vi "DIO_SPI.vi"(0 "DIO.2:0.OUT":fxp<+,3,3> format="%03b", 1 "DIO.2:0.DIR":fxp<+,3,3> format="%03b", 2 "SPI.CNT":u16, 3 "SPI.CNFG":u16 format="%016b", 4 "SPI.DATO":u16, 5 "SPI.GO":T1, 6 "DIO.2/SPI.MOSI Refnum":refnum<k21>, 7 "SELECT.1:0":fxp<+,2,2> format="%02b", 8 "DIO.1/SPI.MISO Refnum":refnum<k21>, 10 "DIO.0/SPI.SCLK Refnum":refnum<k21>) -> (14 "DIO.2:0.IN":fxp<+,3,3> format="%03b", 18 "SPI.DATI":u16, 19 "SPI.STAT":u8 format="%08b")   [LabVIEW 2015]
uses:
  Utilities/Start Boolean.ctl
panel:
  # "SELECT1 | SELECT0 || Functionality\n ---------|---------||------------------\n     0    |    0    || DIO0, DIO1, DIO2\n     0    |    1    || DIO1, SPI: MISO, SCLK (RX Only SPI)\n     1    |    0    || DIO0, SPI: MOSI, SCLK (TX Only SPI)\n     1    |    1    || SPI: MISO, MOSI, SCLK"
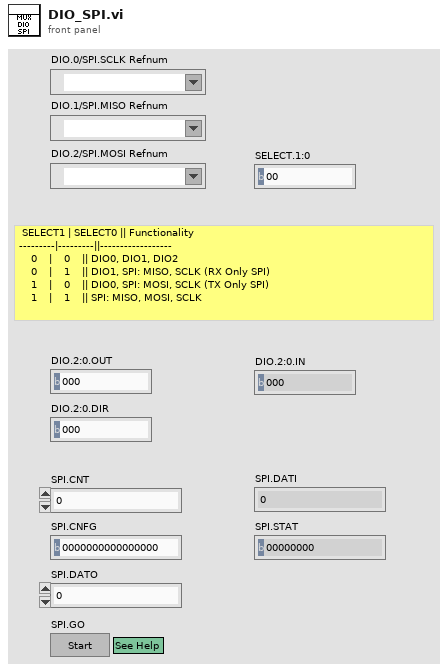
[diagram p1: front panel]
types:
  T1 = typedef "Start Boolean.ctl" = bool
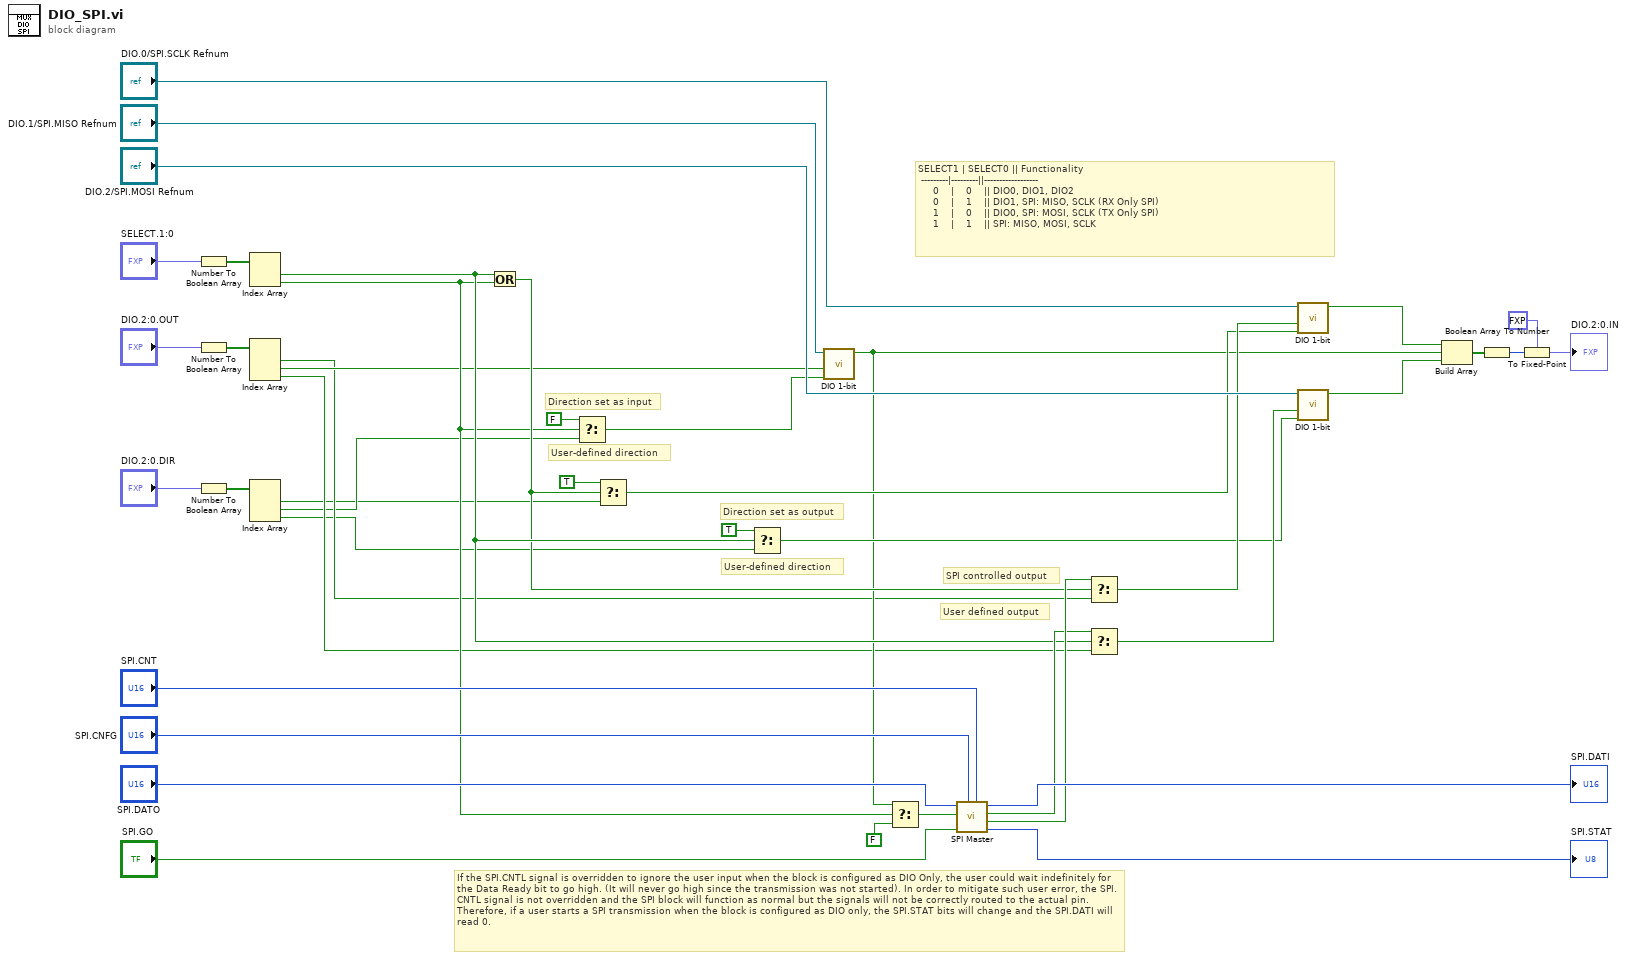
[diagram p0: block diagram]
diagram:
  # "If the SPI.CNTL signal is overridden to ignore the user input when the block is configured as DIO Only, the user could wait indefinitely for the Data Ready bit to go high. (It will never go high since the transmission was not started). In order to mitigate such user error, the SPI.CNTL signal is not overridden and the SPI block will function as normal but the signals will not be correctly routed to the actual pin. Therefore, if a user starts a SPI transmission when the block is configured as DIO only, the SPI.STAT bits will change and the SPI.DATI will read 0."
  # "SELECT1 | SELECT0 || Functionality\n ---------|---------||------------------\n     0    |    0    || DIO0, DIO1, DIO2\n     0    |    1    || DIO1, SPI: MISO, SCLK (RX Only SPI)\n     1    |    0    || DIO0, SPI: MOSI, SCLK (TX Only SPI)\n     1    |    1    || SPI: MISO, MOSI, SCLK"
  # "SPI controlled output"
  # "User defined output"
  # "User-defined direction"
  # "User-defined direction"
  # "Direction set as output"
  # "Direction set as input"
  n1 = Number To Boolean Array(number="SELECT.1:0") -> (Boolean array=w21:bool[])
  n2 = Number To Boolean Array(number="DIO.2:0.OUT") -> (Boolean array=w31:bool[])
  n3 = Number To Boolean Array(number="DIO.2:0.DIR") -> (Boolean array=w28:bool[])
  n4 = Index Array(array=w21) -> (element #1=w12:bool, element #2=w10:bool)  [unwired: 2 in]
  n5 = Index Array(array=w31) -> (element #1=w4:bool, element #2=w6:bool, element #3=w5:bool)  [unwired: 3 in]
  n6 = Index Array(array=w28) -> (element #1=w1:bool, element #2=w3:bool, element #3=w2:bool)  [unwired: 3 in]
  n7 = Or(x=w12, y=w10) -> (x .or. y?=w11:bool)
  n8 = Select(t=FALSE, s=w10, f=w3) -> (s? t:f=w18:bool)
  n9 = Select(t=TRUE, s=w11, f=w1) -> (s? t:f=w17:bool)
  n10 = Select(t=TRUE, s=w12, f=w2) -> (s? t:f=w16:bool)
  n11 = call "DIO 1-bit.vi"("DIR"=w18, "OUT"=w6, "DIO Refnum"="DIO.1/SPI.MISO Refnum") -> ("IN"=w9:bool)  [unwired: 8 in]
  n12 = Select(t=w9, s=w10, f=FALSE) -> (s? t:f=w23:bool)
  n13 = call "SPI Master.vi"("Count"="SPI.CNT", "Configuration"="SPI.CNFG", "Start?"="SPI.GO", "MISO"=w23, "Data Out"="SPI.DATO") -> ("Status"=→"SPI.STAT":u8, "SCLK"=w27:bool, "MOSI"=w25:bool, "Data In"=→"SPI.DATI":u16)  [unwired: 3 in]
  n14 = Select(t=w27, s=w11, f=w4) -> (s? t:f=w26:bool)
  n15 = Select(t=w25, s=w12, f=w5) -> (s? t:f=w24:bool)
  n16 = call "DIO 1-bit.vi"("DIR"=w17, "OUT"=w26, "DIO Refnum"="DIO.0/SPI.SCLK Refnum") -> ("IN"=w8:bool)  [unwired: 8 in]
  n17 = call "DIO 1-bit.vi"("DIR"=w16, "OUT"=w24, "DIO Refnum"="DIO.2/SPI.MOSI Refnum") -> ("IN"=w7:bool)  [unwired: 8 in]
  n18 = Build Array(w8, w9, w7) -> (w19:bool[])
  n19 = Boolean Array To Number(Boolean array=w19) -> (number=w35:u8)
  n20 = To Fixed-Point(fixed-point type=fxp<+,3,3> 0.0 ("DIO0:3.PIN"), number=w35) -> (fixed-point=→"DIO.2:0.IN":fxp<+,3,3>)
